vi "Rinocloud_HTTP_create_folder.vi"(5 "Parent ID":string="name", 6 "Extra metadata array":T1(array[cluster])=[{"Attribute"="", "Value"="", "Data type"=enum."<null>"}], 7 "Notes":string, 8 "Tags":string, 9 "Name":string) -> (0 "body":string, 1 "headers":string, 2 "ID":i32, 3 "Saved":bool)   [LabVIEW 2013]
uses:
  Rinocloud_global_variable.vi
  <vilib>/httpClient/POSTBuffer.vi
  <vilib>/httpClient/LabVIEWHTTPClient.lvlib
panel:
  out "JSON payload":string
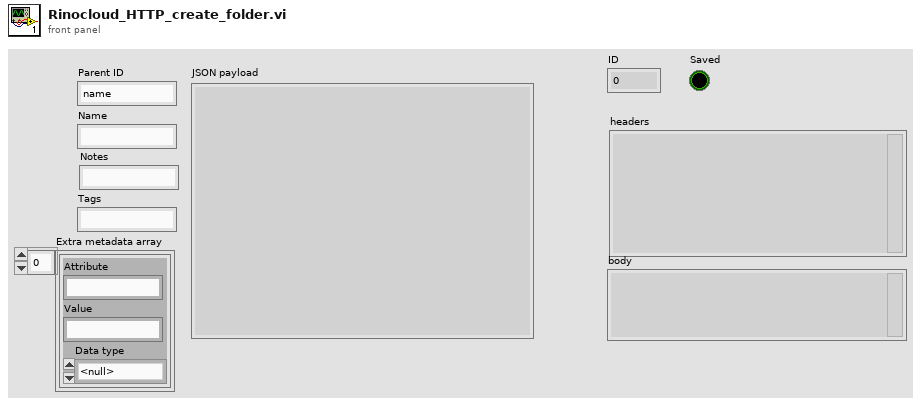
[diagram p1: front panel]
types:
  T1 = cluster{"Attribute":string, "Value":string, "Data type":enum16{"Numeric", "String", "1D array of strings", "1D array of doubles", "Data JSON string", "<null>"}}[]
  T2 = cluster{"Name":string, "Notes":string, "Tags":string}
  T3 = typedef "LabVIEWHTTPClient.lvlib/ClientHandle.ctl" = refnum<k1>
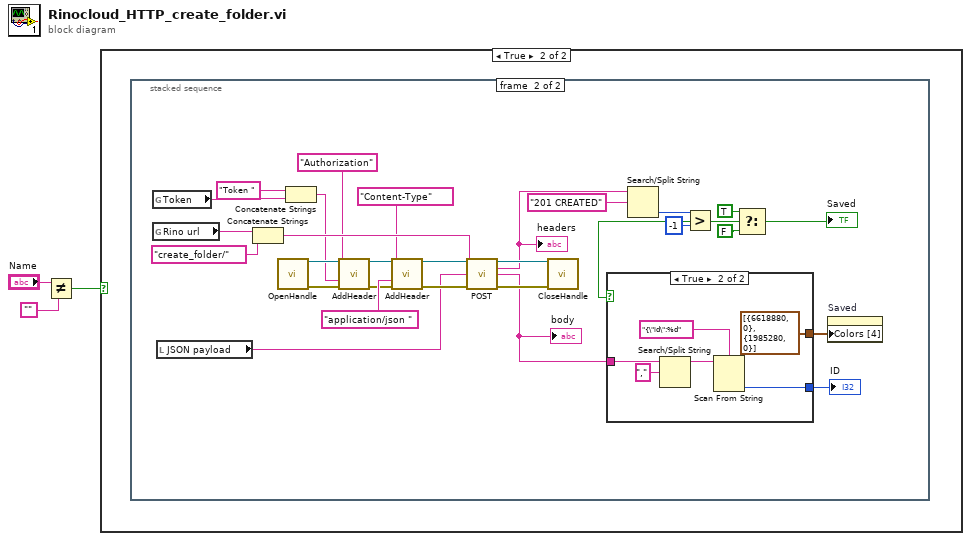
[diagram p0: block diagram]
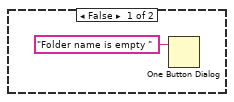
[diagram p2: hidden frame]
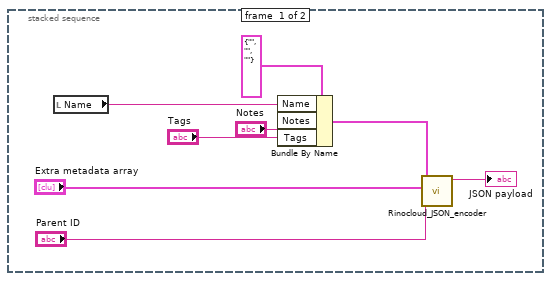
[diagram p3: hidden frame]
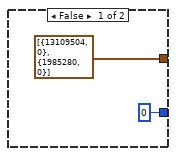
[diagram p4: hidden frame]
diagram:
  n1 = Not Equal?(x="Name", y="") -> (x != y?=w1:bool)
  n2 = case shown="True" w1 {
    frame False {
      n3 = One Button Dialog(message="Folder name is empty ") -> ()  [unwired: 1 in, 1 out]
    }
    frame True {
      n4 = stacked-sequence {
        frame #0 {
          n5 = local read "Name"() -> (w5:string)
          n6 = Bundle By Name(cluster=T2 {"Name"="", "Notes"="", "Tags"=""} ("Metadata"), "Name"=w5, "Notes"="Notes", "Tags"="Tags") -> (w8:T2)
          n7 = call "Rinocloud_JSON_encoder.vi"("parent ID"="Parent ID", "Extra metadata array"="Extra metadata array", "Metadata"=w8) -> ("JSON payload"=→"JSON payload":string)  [unwired: 8 in]
        }
        frame #1 {
          n8 = global read "Rinocloud_global_variable.vi" "Token"() -> (w33:string)
          n9 = global read "Rinocloud_global_variable.vi" "Rino url"() -> (w39:string)
          n10 = local read "JSON payload"() -> (w13:string)
          n11 = Concatenate Strings(w39, "create_folder/" ("Combo Box 2")) -> (w41:string)
          n12 = call <vilib>:"OpenHandle.vi"() -> ("client handle out"=w37:T3, "error out"=w34:errorcluster)  [unwired: 14 in]
          n13 = Concatenate Strings("Token " ("value"), w33) -> (w35:string)
          n14 = call <vilib>:"AddHeader.vi"("client handle"=w37, "header"="Authorization" ("url"), "value"=w35, "error in (no error)"=w34) -> ("client handle out"=w17:T3, "error out"=w15:errorcluster)  [unwired: 10 in]
          n15 = call <vilib>:"AddHeader.vi"("client handle"=w17, "header"="Content-Type", "value"="application/json ", "error in (no error)"=w15) -> ("client handle out"=w16:T3, "error out"=w14:errorcluster)  [unwired: 10 in]
          n16 = call-poly <vilib>:"POST.vi"("client handle"=w16, "url"=w41, "buffer"=w13, "error in (no error)"=w14) -> ("client handle out"=w32:T3, "headers"=w20:string, "body"=w21:string, "error out"=w31:errorcluster)  [unwired: 8 in]
          "headers" <- w20
          "body" <- w21
          n17 = call <vilib>:"CloseHandle.vi"("client handle"=w32, "error in (no error)"=w31) -> ()  [unwired: 13 in, 1 out]
          n18 = Search/Split String(string=w20, search string/char (-)="201 CREATED") -> (offset of match=w29:i32)  [unwired: 1 in, 2 out]
          n19 = Greater?(x=w29, y=-1) -> (0:w27:bool)
          n20 = Select(t=TRUE, s=w27, f=FALSE) -> (s? t:f=w24:bool)
          "Saved" <- w24
          n21 = case shown="True" w24 {
            tunnel: w21 -> [_ w49]
            tunnel: [0 w45] -> w23
            tunnel: [cluster{u32, u32}[] [{13109504, 0}, {1985280, 0}] ("Colors [4]") cluster{u32, u32}[] [{6618880, 0}, {1985280, 0}] ("Colors [4]")] -> w22
            frame False {
            }
            frame True {
              n22 = Search/Split String(string=w49, search string/char (-)=",") -> (substring before match=w47:string)  [unwired: 1 in, 2 out]
              n23 = Scan From String(format string="{\"id\":%d", input string=w47) -> (output 1=w45:i32)  [unwired: 3 in, 3 out]
            }
          }
          "ID" <- w23
          n24 = property on="Saved" class="Bool (strict)"("Colors [4]"=w22) -> ()  [unwired: 2 in, 2 out]
        }
      }
    }
  }
